vi "New GUID.vi"(8 "Error In":errorcluster) -> (0 "Error Out":errorcluster, 3 "GUID":string)   [LabVIEW 2011, in "Tinkerforge.lvlib"]
doc: "This VI generates a Globally Unique Identifier (GUID). The Guid .NET class is used to retrieve the GUID."
uses:
  Tinkerforge.lvlib
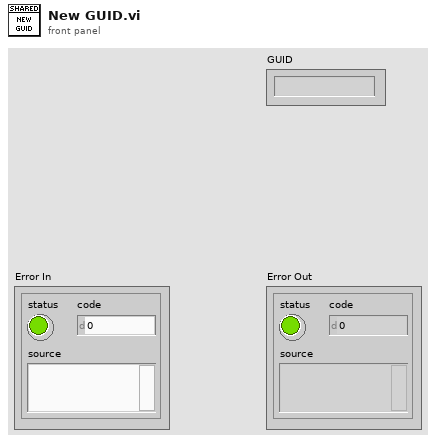
[diagram p1: front panel]
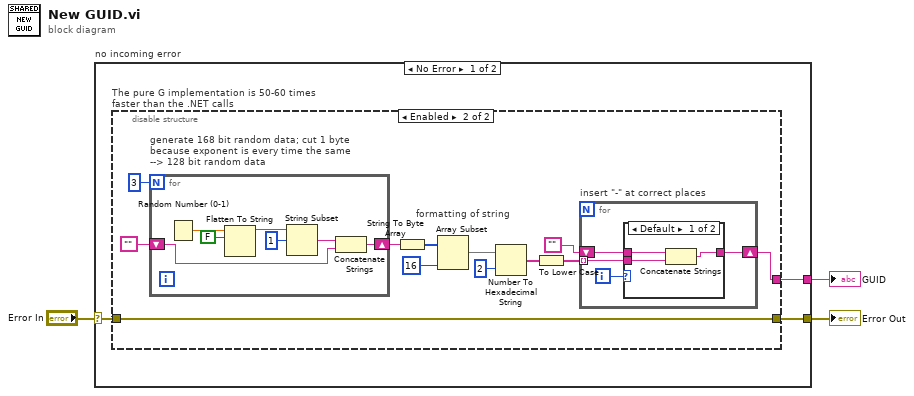
[diagram p0: block diagram]
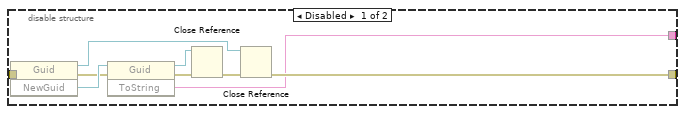
[diagram p2: hidden frame]
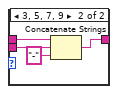
[diagram p3: hidden frame]
diagram:
  n1 = case "no incoming error" shown="No Error" "Error In" {
    selector: "Error In" -> [w6 w46]
    tunnel: [w5 w46] -> w2
    tunnel: [w4 _] -> w1
    frame No Error {
      n2 = disable-structure "The pure G implementation is 50-60 times faster than the .NET calls" shown="Enabled" {
        disable-tunnel: w6 -> [w14 w17]
        disable-tunnel: [w8 w17] -> w5
        disable-tunnel: [w7 w18] -> w4
        frame Disabled {
          n3 = invoke class="Guid" method="NewGuid"(error in=w14) -> (reference out=w9:refnum<k24>, error out=w13:errorcluster, "NewGuid"=w15:refnum<k24>)  [unwired: 2 in]
          n4 = invoke class="Guid" method="ToString"(reference=w15, error in=w13) -> (reference out=w11:refnum<k24>, error out=w12:errorcluster, "ToString"=w7:string)  [unwired: 1 in]
          n5 = Close Reference(reference=w11, error in (no error)=w12) -> (error out=w10:errorcluster)
          n6 = Close Reference(reference=w9, error in (no error)=w10) -> (error out=w8:errorcluster)
        }
        frame Enabled {
          # "formatting of string"
          n7 = for "generate 168 bit random data; cut 1 byte\nbecause exponent is every time the same\n--> 128 bit random data" {
            N: 3 -> [_]
            shift-right: [w41] -> w20
            shift-left: "" -> [w40]
            n8 = Random Number (0-1)() -> (number: 0 to 1=w45:dbl)
            n9 = Flatten To String(anything=w45, prepend array or string size? (T)=FALSE) -> (data string=w44:string)  [unwired: 2 in, 2 out]
            n10 = String Subset(string=w44, offset (0)=1) -> (substring=w43:string)  [unwired: 1 in]
            n11 = Concatenate Strings(w43, w40) -> (w41:string)
          }
          n12 = String To Byte Array(string=w20) -> (unsigned byte array=w25:u8[])
          n13 = Array Subset(array=w25, length=16) -> (w23:u8[])  [unwired: 1 in]
          n14 = Number To Hexadecimal String(1:i16 2 ("width (-)"), 2:w23) -> (0:w21:string[])
          n15 = To Lower Case(string=w21) -> (all lower case string=w19:string[])
          n16 = for "insert \"-\" at correct places" {
            tunnel: w19 -> [w30] mode=indexing
            shift-right: [w28] -> w18
            shift-left: "" -> [w29]
            i -> [w31]
            n17 = case shown="Default" w31 {
              tunnel: w30 -> [w33 w37]
              tunnel: w29 -> [w34 w38]
              tunnel: [w32 w36] -> w28
              frame Default {
                n18 = Concatenate Strings(w34, w33) -> (w32:string)
              }
              frame 3, 5, 7, 9 {
                n19 = Concatenate Strings(w38, w37, "-" ("string")) -> (w36:string)
              }
            }
          }
        }
      }
    }
    frame Error {
    }
  }
  "Error Out" <- w2
  "GUID" <- w1
